vi "Reset Device Core.vi"(8 "error in (no error)":errorcluster, 11 "BNT_DAQmx-MCSV in":refnum<class "BNT_DAQmx-MCSV.lvclass">) -> (0 "error out":errorcluster, 3 "BNT_DAQmx-MCSV out":refnum<class "BNT_DAQmx-MCSV.lvclass">)   [LabVIEW 2017, in "BNT_DAQmx.lvlib" / "BNT_DAQmx-MCSV.lvclass"]
doc: "Perform reset of device."
uses:
  BNT_DAQmx-MCSV.lvclass
  C:/User/Brand/LVP/TASCA/UTCS/Packages/CSPP_Core/Actors/CSPP_DeviceActor/CSPP_DeviceActor.lvclass
  CSPP_Core/Actors/CSPP_DeviceActor/CSPP_DeviceActor.lvclass
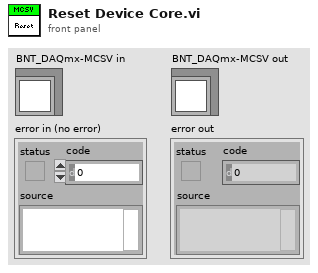
[diagram p1: front panel]
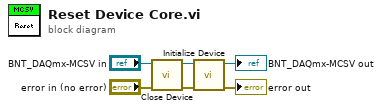
[diagram p0: block diagram]
diagram:
  n1 = call "Close Device.vi"("error in (no error)"="error in (no error)", "CSPP_DeviceActor in"="BNT_DAQmx-MCSV in") -> ("error out"=w4:errorcluster, "CSPP_DeviceActor out"=w3:refnum<class "BNT_DAQmx-MCSV.lvclass">)  [unwired: 8 in]
  n2 = call "Initialize Device.vi"("error in (no error)"=w4, "CSPP_DeviceActor in"=w3) -> ("error out"=→"error out":errorcluster, "CSPP_DeviceActor out"=→"BNT_DAQmx-MCSV out":refnum<class "BNT_DAQmx-MCSV.lvclass">)  [unwired: 8 in]
